vi "Pump Output in Procent.vi"(11 "Cluster.Pump Concentrations-Cluster":T1 caption="Pump Output in") -> (3 "Pump Output out":T1)   [LabVIEW 2020, in "Linearisierung v2.lvlib" / "Gasteiler.lvlib" / "HovaCAL_Interface.lvlib" / "Helper.lvlib"]
uses:
  Helper.lvlib
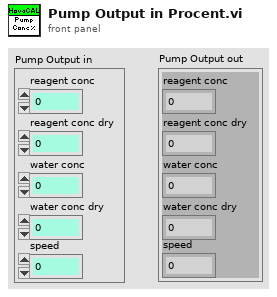
[diagram p1: front panel]
types:
  T1 = cluster{"reagent conc":dbl, "reagent conc dry":dbl, "water conc":dbl, "water conc dry":dbl, "speed":dbl}
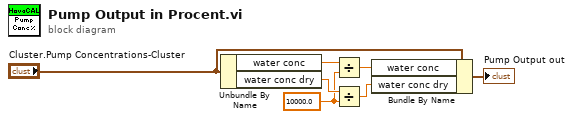
[diagram p0: block diagram]
diagram:
  w1 = 10000.0 ("y")
  n1 = Unbundle By Name("Cluster.Pump Concentrations-Cluster") -> ("water conc"=w7:dbl, "water conc dry"=w3:dbl)
  n2 = Divide(x=w7, y=w1) -> (x/y=w4:dbl)
  n3 = Divide(x=w3, y=w1) -> (x/y=w2:dbl)
  n4 = Bundle By Name(cluster="Cluster.Pump Concentrations-Cluster", "water conc"=w4, "water conc dry"=w2) -> (→"Pump Output out":T1)
